vi "Error to Spreadsheet.vi"() -> ()   [LabVIEW 2014]
uses:
  <vilib>/Platform/TimedLoop/XDataNode/timing_clust.ctl
  <vilib>/Platform/TimedLoop/XDataNode/nitl_modes.ctl
  <vilib>/Platform/TimedLoop/XDataNode/wakeup.ctl
  <vilib>/Utility/file.llb/Write To Spreadsheet File (string).vi
  <vilib>/platform/TimedLoop/XDataNode/XDataNode.xnode
  <vilib>/Platform/TimedLoop/XDataNode/XDNodeRunTimeDep.lvlib
panel:
  in  "error in (no error)":errorcluster
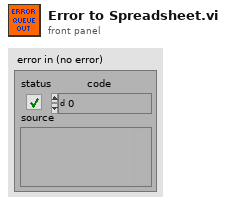
[diagram p1: front panel]
types:
  T1 = typedef "XDNodeRunTimeDep.lvlib/timing_clust.ctl" = cluster{"Expected End [f-1]":u64, "Actual End [f-1]":u64, "Finished Late? [f-1]":bool, "Expected End [i-1]":u64, "Actual End [i-1]":u64, "Finished Late? [i-1]":bool, "Expected Start [i]":u64, "Actual Start [i]":u64, "Expected Start [f]":u64, "Actual Start [f]":u64, "Source Name":string, "Structure Name":string, "Period":i64, "Deadline":i64, "Offset":i64, "Start":i64, "Priority":i32, "Timeout":i32, "Mode":T2, "Wakeup Reason":T3, "Error":errorcluster, "Source Type":string, "Secondary Source Type":string, "Global End Time":u64, "Global Start Time":u64, "Frame Duration":u64, "Iteration Duration":u64, "Assigned CPU":i32, "I/O Scan Engine Mode":u32}
  T2 = typedef "XDNodeRunTimeDep.lvlib/nitl_modes.ctl" = enum32{"No Change", "Process missed periods, maintain original phase", "Discard missed periods, maintain original phase", "Process missed periods, ignore original phase", "Discard missed periods, ignore original phase"}
  T3 = typedef "XDNodeRunTimeDep.lvlib/wakeup.ctl" = enum32{"Normal", "Aborted", "Asynchronous wakeup", "Timing source error", "Timed loop error", "Timeout"}
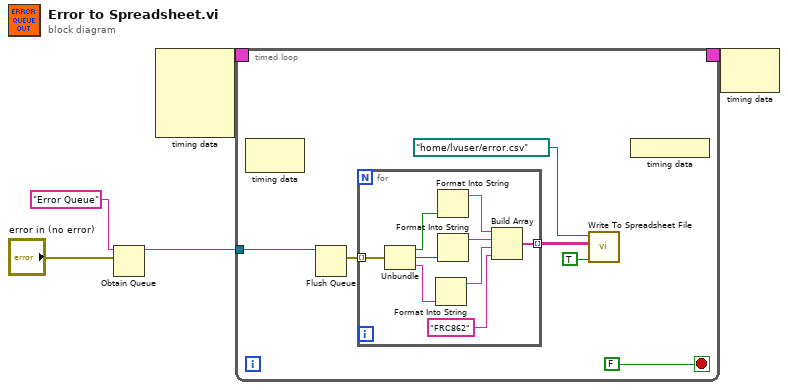
[diagram p0: block diagram]
diagram:
  n1 = Obtain Queue(name (unnamed)="Error Queue", element data type="error in (no error)") -> (queue out=w3:refnum<queue>)  [unwired: 3 in, 2 out]
  n2 = node-c288() -> (w2:T1)  [unwired: 4 in]
  n3 = timed-loop {
    tunnel: w3 -> [w7]
    timing: w2 -> [_]
    timing-out: [_] -> w1
    stop <- FALSE stop-if-true
    n4 = node-c288() -> ()  [unwired: 1 in, 1 out]
    n5 = Flush Queue(queue=w7) -> (remaining elements=w10:errorcluster[])  [unwired: 1 in, 2 out]
    n6 = for {
      tunnel: w10 -> [w22] mode=indexing
      tunnel: [w15] -> w6 mode=indexing
      n7 = Unbundle(w22) -> ("status"=w21:bool, "code"=w20:i32, "source"=w19:string)
      n8 = Format Into String(w19) -> (resulting string=w16:string)  [unwired: 3 in, 1 out]
      n9 = Format Into String(w21) -> (resulting string=w18:string)  [unwired: 3 in, 1 out]
      n10 = Format Into String(w20) -> (resulting string=w17:string)  [unwired: 3 in, 1 out]
      n11 = Build Array(w18, w17, w16, "FRC862" ("element")) -> (w15:string[])
    }
    n12 = call-poly <vilib>:"Write To Spreadsheet File.vi"("append to file? (new file:F)"=TRUE, "2D data"=w6, "file path (dialog if empty)"=path "/home/lvuser/error.csv" ("file path")) -> ()  [unwired: 5 in, 1 out]
    n13 = node-c288() -> ()  [unwired: 1 out]
  }
  n14 = node-c288(w1) -> ()  [unwired: 1 out]
